vi "Start Sync.vi"(8 "error in (no error)":errorcluster, 11 "gRPC service in":refnum<class "OOBgRPCService.lvclass">) -> (0 "error out":errorcluster, 3 "gRPC service out":refnum<class "OOBgRPCService.lvclass">)   [LabVIEW 2025, in "OOB gRPC Server.lvlib" / "OOBgRPCService.lvclass"]
uses:
  OOBgRPCService.lvclass
  OOBgRPCService.lvclass/OOBgRPCService.ctl
  OOB Data Transfer/OOB Data Transfer.lvlib
  RPC Messages/hwval_GenericResponse.ctl
  OOB gRPC Server.lvlib
  RPC Messages/hwval_StatusResponse.ctl
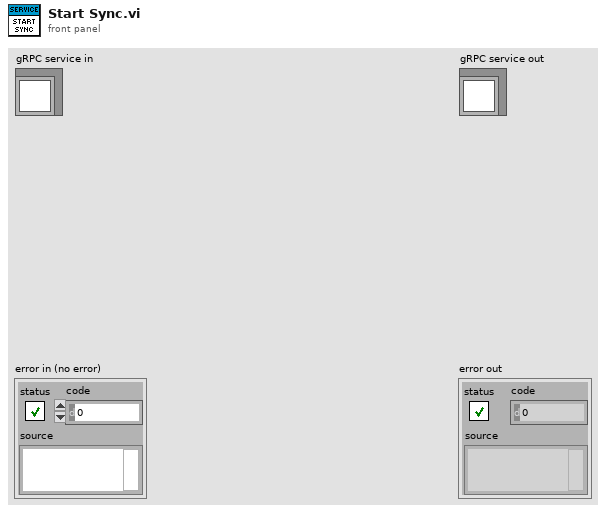
[diagram p1: front panel]
types:
  T1 = typedef "OOB gRPC Server.lvlib/hwval_GenericResponse.ctl" = cluster{"Payload":u8[]}
  T2 = typedef "OOB gRPC Server.lvlib/hwval_StatusResponse.ctl" = cluster{"Status":bool, "Code":i32, "Message":string}
  T3 = typedef "OOB gRPC Server.lvlib/OOBgRPCService.lvclass/Server Internal UEs.ctl" = cluster{"OOBgRPCService Generic Internal UE":refnum<user-event>, "OOBgRPCService PauseResume Internal UE":refnum<user-event>, "OOBgRPCService Export Internal UE":refnum<user-event>}
  T4 = typedef "OOB gRPC Server.lvlib/OOBgRPCService.lvclass/Server gRPC UEs.ctl" = cluster{"OOBgRPCService Generic gRPC UE":refnum<user-event>, "OOBgRPCService PauseResume gRPC UE":refnum<user-event>, "OOBgRPCService Export gRPC UE":refnum<user-event>}
  T5 = typedef "grpc-lvsupport-release.lvlib/grpcId.ctl" = u64
  T6 = typedef "OOB gRPC Server.lvlib/hwval_GenericRequest.ctl" = cluster{"Command":string, "Payload":u8[]}
  T7 = typedef "OOB Data Transfer.lvlib/OOB to Logic Data.ctl" = cluster{"PauseResume":bool, "Export":string, "Double":dbl, "String":string}
  T8 = typedef "OOB gRPC Server.lvlib/hwval_BoolRequest.ctl" = cluster{"BooleanData":bool}
  T9 = typedef "OOB gRPC Server.lvlib/hwval_ExportRequest.ctl" = cluster{"FileType":string}
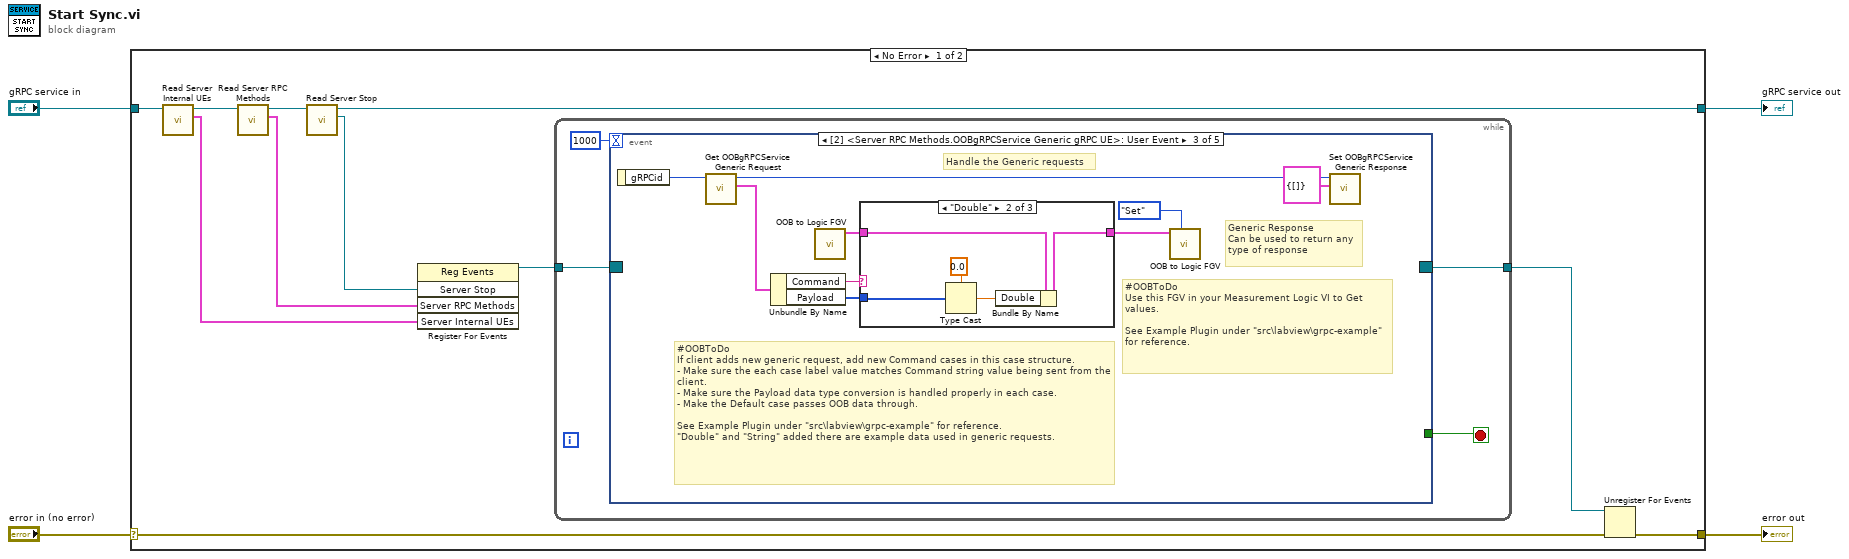
[diagram p0: block diagram]
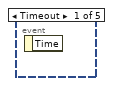
[diagram p2: hidden frame]
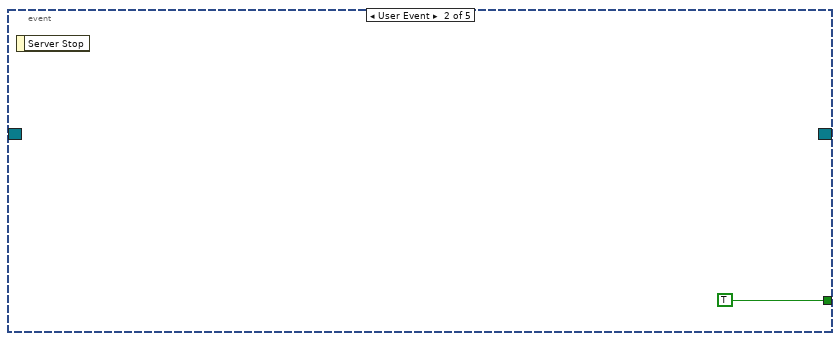
[diagram p3: hidden frame]
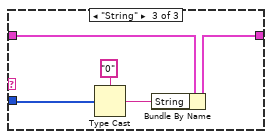
[diagram p5: hidden frame]
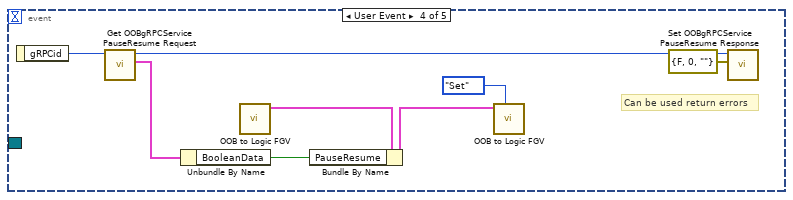
[diagram p6: hidden frame]
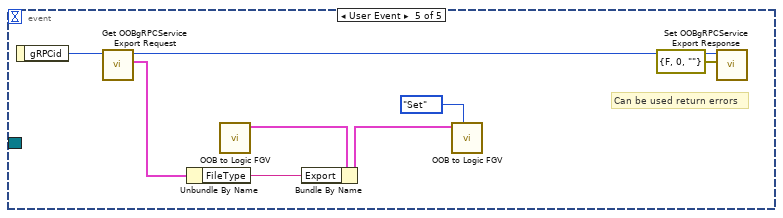
[diagram p7: hidden frame]
diagram:
  n1 = case shown="No Error" "error in (no error)" {
    selector: "error in (no error)" -> [w9 w58]
    tunnel: [w8 w58] -> w3
    tunnel: [w6 w57] -> w1
    tunnel: "gRPC service in" -> [w15 w57]
    frame No Error {
      n2 = call "Read Server Internal UEs.vi"("gRPC service in"=w15) -> ("Server Internal UEs"=w13:T3, "gRPC service out"=w14:refnum<class "OOBgRPCService.lvclass">)  [unwired: 8 in, 1 out]
      n3 = call "Read Server RPC Methods.vi"("gRPC service in"=w14) -> ("Server RPC Methods"=w7:T4, "gRPC service out"=w12:refnum<class "OOBgRPCService.lvclass">)  [unwired: 8 in, 1 out]
      n4 = call-dynamic "Read Server Stop.vi"("gRPC service in"=w12) -> ("Server Stop"=w5:refnum<user-event>, "gRPC service out"=w6:refnum<class "OOBgRPCService.lvclass">)  [unwired: 8 in, 1 out]
      n5 = register-events(w5, w7, w13) -> (reference out=w11:refnum<event-registration>)  [unwired: 2 in, 1 out]
      n6 = while {
        tunnel: w11 -> [w19]
        tunnel: [w17] -> w10
        stop <- w18 stop-if-true
        n7 = event "RPC Methods Event Structure" shown="[2] <Server RPC Methods.OOBgRPCService Generic gRPC UE>: User Event" {
          selector: w19 -> [_ _ _ _ _]
          dyn-events: [_ _ _ _ _] -> w17
          timeout: 1000 -> [_ _ _ _ _]
          tunnel: [_ TRUE _ _ _] -> w18
          event Timeout {
            n8 = event-data() -> ()  [unwired: 1 in, 1 out]
          }
          event User Event {
            n9 = event-data() -> ()  [unwired: 1 in, 1 out]
          }
          event User Event {
            # "#OOBToDo \nIf client adds new generic request, add new Command cases in this case structure. \n- Make sure the each case label value matches Command string value being sent from the client.\n- Make sure the Payload data type conversion is handled properly in each case.\n- Make the Default case passes OOB data through.\n\nSee Example Plugin under \"src\\labview\\grpc-example\" for reference. \n\"Double\" and \"String\" added there are example data used in generic requests."
            # "Handle the Generic requests"
            # "Generic Response\nCan be used to return any type of response"
            # "#OOBToDo \nUse this FGV in your Measurement Logic VI to Get values.\n\nSee Example Plugin under \"src\\labview\\grpc-example\" for reference."
            n10 = event-data() -> ("gRPCid"=w29:T5)  [unwired: 1 in]
            n11 = call "Get OOBgRPCService Generic Request.vi"("gRPCid"=w29) -> ("Message Data"=w27:T6, "gRPCid out"=w28:T5)  [unwired: 8 in, 1 out]
            n12 = Unbundle By Name(w27) -> ("Command"=w22:string, "Payload"=w21:u8[])
            n13 = call "OOB to Logic FGV.vi"() -> ("OOB to Logic Data out"=w24:T7)  [unwired: 10 in, 1 out]
            n14 = case shown="\"Double\"" w22 {
              tunnel: w24 -> [w30 w35 w40]
              tunnel: [w30 w34 w39] -> w23
              tunnel: w21 -> [_ w31 w36]
              frame Default {
              }
              frame "Double" {
                n15 = Type Cast(type=0.0 ("Double"), x=w31) -> (*(type *) &x=w33:dbl)
                n16 = Bundle By Name(cluster=w35, "Double"=w33) -> (w34:T7)
              }
              frame "String" {
                n17 = Type Cast(type="0" ("Double"), x=w36) -> (*(type *) &x=w38:string)
                n18 = Bundle By Name(cluster=w40, "String"=w38) -> (w39:T7)
              }
            }
            n19 = call "OOB to Logic FGV.vi"("Op (Get)"=enum16{"Get", "Set"}."Set", "OOB to Logic Data in"=w23) -> ()  [unwired: 8 in, 2 out]
            n20 = call "Set OOBgRPCService Generic Response.vi"("Message Data"=T1 {"Payload"=[]}, "gRPCid in"=w28) -> ()  [unwired: 9 in, 1 out]
          }
          event User Event {
            # "Can be used return errors"
            n21 = event-data() -> ("gRPCid"=w42:T5)  [unwired: 1 in]
            n22 = call "Get OOBgRPCService PauseResume Request.vi"("gRPCid"=w42) -> ("Message Data"=w44:T8, "gRPCid out"=w45:T5)  [unwired: 8 in, 1 out]
            n23 = Unbundle By Name(w44) -> ("BooleanData"=w43:bool)
            n24 = call "OOB to Logic FGV.vi"() -> ("OOB to Logic Data out"=w47:T7)  [unwired: 10 in, 1 out]
            n25 = Bundle By Name(cluster=w47, "PauseResume"=w43) -> (w46:T7)
            n26 = call "OOB to Logic FGV.vi"("Op (Get)"=enum16{"Get", "Set"}."Set", "OOB to Logic Data in"=w46) -> ()  [unwired: 8 in, 2 out]
            n27 = call "Set OOBgRPCService PauseResume Response.vi"("Message Data"=T2 {"Status"=FALSE, "Code"=0, "Message"=""}, "gRPCid in"=w45) -> ()  [unwired: 9 in, 1 out]
          }
          event User Event {
            # "Can be used return errors"
            n28 = event-data() -> ("gRPCid"=w50:T5)  [unwired: 1 in]
            n29 = call "Get OOBgRPCService Export Request.vi"("gRPCid"=w50) -> ("Message Data"=w52:T9, "gRPCid out"=w56:T5)  [unwired: 8 in, 1 out]
            n30 = Unbundle By Name(w52) -> ("FileType"=w51:string)
            n31 = call "OOB to Logic FGV.vi"() -> ("OOB to Logic Data out"=w54:T7)  [unwired: 10 in, 1 out]
            n32 = Bundle By Name(cluster=w54, "Export"=w51) -> (w53:T7)
            n33 = call "OOB to Logic FGV.vi"("Op (Get)"=enum16{"Get", "Set"}."Set", "OOB to Logic Data in"=w53) -> ()  [unwired: 8 in, 2 out]
            n34 = call "Set OOBgRPCService Export Response.vi"("Message Data"=T2 {"Status"=FALSE, "Code"=0, "Message"=""}, "gRPCid in"=w56) -> ()  [unwired: 9 in, 1 out]
          }
        }
      }
      n35 = Unregister For Events(event registration refnum=w10, error in=w9) -> (error out=w8:errorcluster)
    }
    frame Error {
    }
  }
  "error out" <- w3
  "gRPC service out" <- w1
